vi "Configure.vi"(8 "error in (no error)":errorcluster, 11 "GRMActor in":refnum<class "MicroscopeController.lvclass">) -> (0 "error out":errorcluster, 3 "GRMActor out":refnum<class "MicroscopeController.lvclass">)   [LabVIEW 2020, in "MicroscopeController.lvlib" / "MicroscopeController.lvclass"]
uses:
  MicroscopeController.lvclass
  MicroscopeController.lvclass/MicroscopeController.ctl
  Model/Hardware Abstraction Layer/Component/GenericActor/GenericActor/GenericController.lvclass
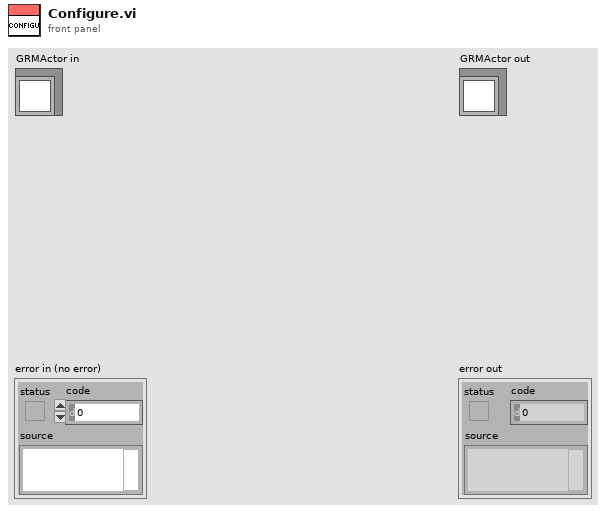
[diagram p1: front panel]
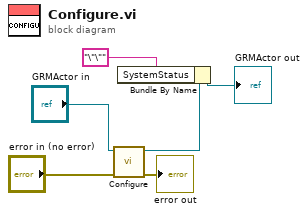
[diagram p0: block diagram]
diagram:
  n1 = call-parent "Configure.vi"("error in (no error)"="error in (no error)", "GRMActor in"="GRMActor in") -> ("error out"=→"error out":errorcluster, "GRMActor out"=w5:refnum<class "MicroscopeController.lvclass">)  [unwired: 8 in]
  n2 = Bundle By Name(cluster=w5, "SystemStatus"="\"\"") -> (→"GRMActor out":refnum<class "MicroscopeController.lvclass">)
